vi "GetAndSetEventSize.vi"(8 "error in (no error)":errorcluster, 10 "Override Max Event size (Data rate bytes/s). Use MIDAS Default = 0":u32, 11 "DataPacker in":refnum<class "DataPacker.lvclass">) -> (0 "error out":errorcluster, 2 "Log Client info (non fatal)":errorcluster, 3 "DataPacker out":refnum<class "DataPacker.lvclass">)   [LabVIEW 2018, in "feGEM DataPacker.lvlib"]
uses:
  feGEM DataPacker.lvlib
  DataPacker.lvclass
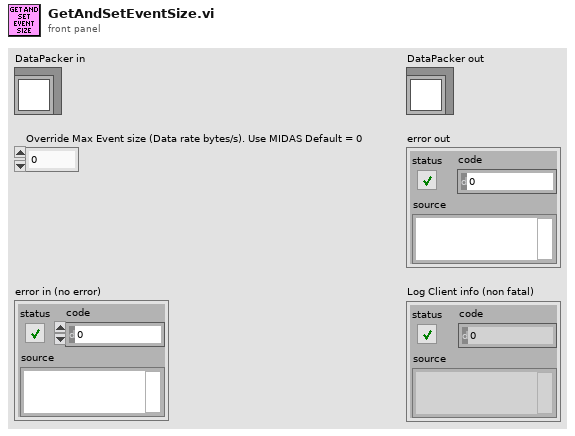
[diagram p1: front panel]
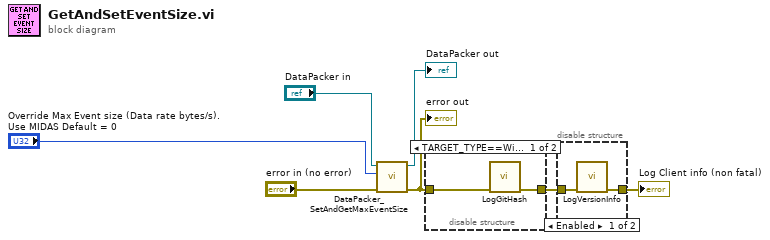
[diagram p0: block diagram]
diagram:
  n1 = call "DataPacker_SetAndGetMaxEventSize.vi"("error in (no error)"="error in (no error)", "Set Event Max Size"="Override Max Event size (Data rate bytes/s). Use MIDAS Default = 0", "DataPacker in"="DataPacker in") -> ("error out"=w7:errorcluster, "DataPacker out"=→"DataPacker out":refnum<class "DataPacker.lvclass">)  [unwired: 7 in]
  "error out" <- w7
  n2 = disable-structure shown="TARGET_TYPE==Windows" {
    disable-tunnel: w7 -> [w9 w10]
    disable-tunnel: [w8 w10] -> w6
    frame condition #0 (active) {
      n3 = call "LogGitHash.vi"("error in (no error)"=w9) -> ("error out"=w8:errorcluster)  [unwired: 10 in]
    }
    frame condition #1 {
    }
  }
  n4 = disable-structure shown="Enabled" {
    disable-tunnel: w6 -> [w12 w13]
    disable-tunnel: [w11 w13] -> w5
    frame Enabled {
      n5 = call "LogVersionInfo.vi"("error in (no error)"=w12) -> ("error out"=w11:errorcluster)  [unwired: 10 in]
    }
    frame Disabled {
    }
  }
  "Log Client info (non fatal)" <- w5
